vi "Progetto Sistemi Di Acquisizione Dati Urzino Davide.vi"() -> ()   [LabVIEW 2015]
uses:
  <vilib>/Instr/_visa.llb/VISA Configure Serial Port (Instr).vi
  <vilib>/smtpClient/Set Message Text.vi
  <vilib>/smtpClient/LabVIEWSMTPClient.lvlib
panel:
  in  "Invia Mail":bool
  in  "Percorso File":path
  out "ora corrente":string
  out "data corrente":string
  out "ora accensione":string
  out "data accensione":string
  out "Pulsante premuto":bool
  out "Contatore Pulsante":i32
  out "Grafico lettura fotodiodo":cluster{"Value":dbl, "Value":dbl}(graph)
  in  "stop":bool
  in  "Impostazione \nSoglia":dbl
  out "Soglia superata":bool
  out "Contatore Pezzi":i32
  out "Lettura bottone da seriale":string
  out "Lettura fotodiodo da seriale":dbl
  out "Minuto passato":bool
  # "Data e Ora di Start"
  # "Data e Ora Correnti"
  # "Imposta \nSoglia"
  # "Contatore Pezzi"
  # "Contatore Pulsante"
  # "Pulsante Premuto"
  # "Soglia Superata"
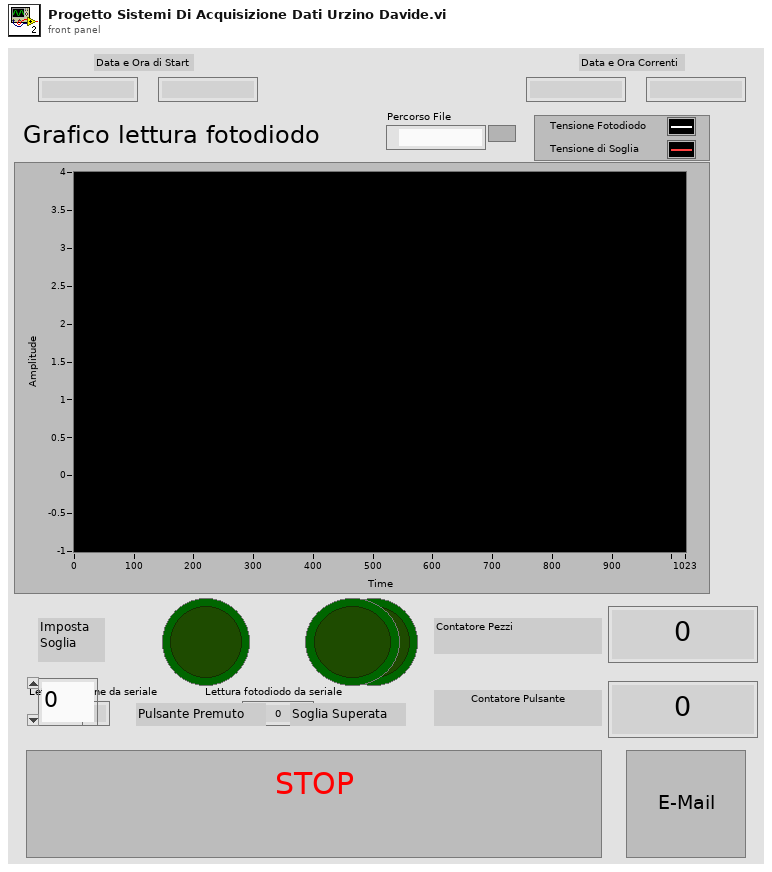
[diagram p1: front panel]
types:
  T1 = enum16{"open", "replace", "create", "open or create", "replace or create", "replace or create with confirmation"}
  T2 = typedef "LabVIEWSMTPClient.lvlib/SmtpClientHandle.ctl" = refnum<k1>
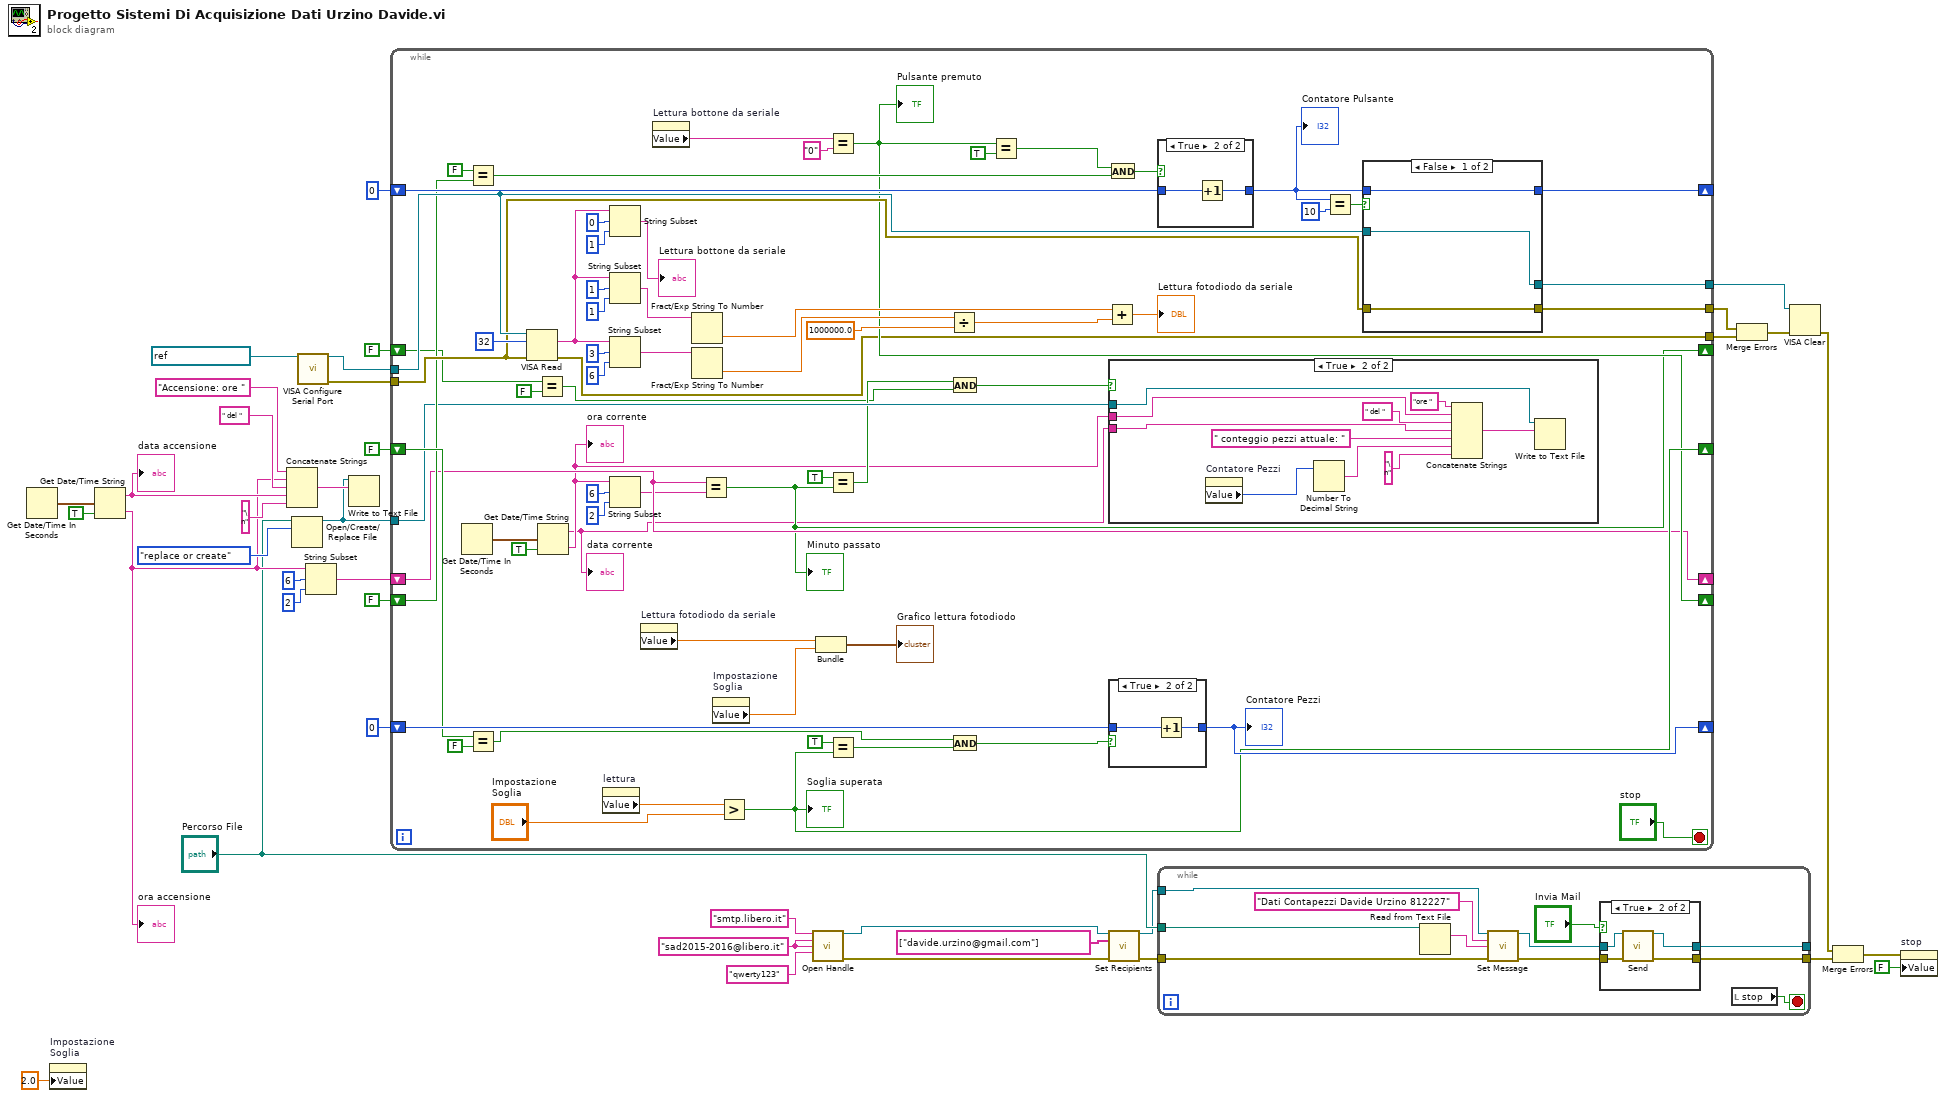
[diagram p0: block diagram]
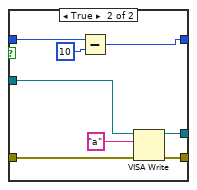
[diagram p4: hidden frame]
diagram:
  w7 = "sad2015-2016@libero.it" ("from")
  n1 = Get Date/Time In Seconds() -> (seconds since 1Jan1904=w31:timestamp)
  n2 = property on="Impostazione \nSoglia" class="DigNum (strict)"("Value"=2.0 ("Impostazione \nSoglia")) -> ()  [unwired: 2 in, 2 out]
  n3 = Get Date/Time String(seconds (now)=w31, want seconds? (F)=TRUE) -> (date string=w26:string, time string=w22:string)  [unwired: 1 in]
  "data accensione" <- w26
  "ora accensione" <- w22
  n4 = Concatenate Strings("Accensione: ore " ("string"), w22, " del " ("string"), w26, "\n" ("string")) -> (w29:string)
  n5 = Open/Create/Replace File(file path (use dialog)="Percorso File", operation (0:open)=T1."replace or create") -> (refnum out=w19:refnum<file>)  [unwired: 4 in, 2 out]
  n6 = call-poly "VISA Configure Serial Port"("VISA resource name"=refnum<visa-resource-name> "ASRL5::INSTR") -> ("VISA resource name out"=w39:refnum<visa-resource-name>, "error out"=w37:errorcluster)  [unwired: 13 in]
  n7 = String Subset(string=w22, offset (0)=6, length (rest)=2 ("length (rest)")) -> (substring=w21:string)
  n8 = Write to Text File(file (use dialog)=w19, text=w29) -> ()  [unwired: 2 in, 3 out]
  n9 = while {
    tunnel: w39 -> [w76]
    tunnel: w37 -> [w75]
    shift-right: [w73] -> _
    shift-left: 0 -> [w104]
    shift-right: [w70] -> _
    shift-left: FALSE -> [w72]
    shift-right: [w74] -> _
    shift-left: 0 -> [w79]
    shift-right: [w59] -> _
    shift-left: FALSE ("x") -> [w66]
    tunnel: w19 -> [w56]
    shift-right: [w53] -> _
    shift-left: w21 -> [w53]
    shift-right: [w45] -> _
    shift-left: FALSE ("want seconds? (F)") -> [w50]
    tunnel: [w42] -> w16
    tunnel: [w41] -> w15
    tunnel: [w40] -> w14
    stop <- "stop" stop-if-true
    n10 = Get Date/Time In Seconds() -> (seconds since 1Jan1904=w58:timestamp)
    n11 = Equal?(x=FALSE, y=w66) -> (x = y?=w62:bool)
    n12 = Equal?(x=w72, y=FALSE) -> (x = y?=w67:bool)
    n13 = VISA Read(VISA resource name=w76, byte count=u32 32, error in (no error)=w75) -> (read buffer=w83:string, error out=w41:errorcluster)  [unwired: 2 out]
    n14 = Equal?(x=w50, y=FALSE ("want seconds? (F)")) -> (x = y?=w47:bool)
    n15 = Get Date/Time String(seconds (now)=w58, want seconds? (F)=TRUE) -> (date string=w43:string, time string=w44:string)  [unwired: 1 in]
    "data corrente" <- w43
    "ora corrente" <- w44
    n16 = property on="lettura" class="DigNum (strict)"() -> ("Value"=w92:dbl)  [unwired: 2 in, 2 out]
    n17 = String Subset(string=w83, offset (0)=0, length (rest)=1 ("length (rest)")) -> (substring=→"Lettura bottone da seriale":string)
    n18 = String Subset(string=w83, offset (0)=1, length (rest)=1 ("length (rest)")) -> (substring=w102:string)
    n19 = String Subset(string=w83, offset (0)=3, length (rest)=6 ("length (rest)")) -> (substring=w100:string)
    n20 = String Subset(string=w44, offset (0)=6, length (rest)=2 ("length (rest)")) -> (substring=w52:string)
    n21 = property on="Lettura fotodiodo da seriale" class="DigNum (strict)"() -> ("Value"=w89:dbl)  [unwired: 2 in, 2 out]
    n22 = property on="Lettura bottone da seriale" class="Str"() -> ("Value"=w81:string)  [unwired: 2 in, 2 out]
    n23 = Fract/Exp String To Number(string=w102) -> (number=w97:dbl)  [unwired: 3 in, 1 out]
    n24 = Fract/Exp String To Number(string=w100) -> (number=w99:dbl)  [unwired: 3 in, 1 out]
    n25 = Equal?(x=w53, y=w52) -> (x = y?=w45:bool)
    "Minuto passato" <- w45
    n26 = property on="Impostazione \nSoglia" class="DigNum (strict)"() -> ("Value"=w88:dbl)  [unwired: 2 in, 2 out]
    n27 = Greater?(x=w92, y="Impostazione \nSoglia") -> (0:w70:bool)
    "Soglia superata" <- w70
    n28 = Bundle("Value"=w89, "Value"=w88) -> (→"Grafico lettura fotodiodo":cluster{"Value":dbl, "Value":dbl})  [unwired: 1 in]
    n29 = Equal?(x=w81, y="0") -> (x = y?=w59:bool)
    "Pulsante premuto" <- w59
    n30 = Equal?(x=TRUE, y=w45) -> (x = y?=w48:bool)
    n31 = Equal?(x=TRUE, y=w70) -> (x = y?=w68:bool)
    n32 = Divide(x=w99, y=1000000.0) -> (x/y=w96:dbl)
    n33 = And(x=w48, y=w47) -> (x .and. y?=w46:bool)
    n34 = And(x=w67, y=w68) -> (x .and. y?=w86:bool)
    n35 = Equal?(x=w59, y=TRUE) -> (x = y?=w63:bool)
    n36 = Add(x=w97, y=w96) -> (x+y=→"Lettura fotodiodo da seriale":dbl)
    n37 = And(x=w63, y=w62) -> (x .and. y?=w61:bool)
    n38 = case shown="True" w46 {
      tunnel: w56 -> [_ w115]
      tunnel: w44 -> [_ w112]
      tunnel: w43 -> [_ w110]
      frame False {
      }
      frame True {
        n39 = property on="Contatore Pezzi" class="DigNum (strict)"() -> ("Value"=w107:i32)  [unwired: 2 in, 2 out]
        n40 = Number To Decimal String(number=w107) -> (decimal integer string=w106:string)  [unwired: 1 in]
        n41 = Concatenate Strings("ore " ("string"), w112, " del " ("string"), w110, " conteggio pezzi attuale: " ("string"), w106, "\n" ("string")) -> (w114:string)
        n42 = Write to Text File(file (use dialog)=w115, text=w114) -> ()  [unwired: 2 in, 3 out]
      }
    }
    n43 = case shown="True" w86 {
      tunnel: w104 -> [w130 w132]
      tunnel: [w130 w131] -> w73
      frame False {
      }
      frame True {
        n44 = Increment(x=w132) -> (x+1=w131:i32)
      }
    }
    "Contatore Pezzi" <- w73
    n45 = case shown="True" w61 {
      tunnel: w79 -> [w127 w128]
      tunnel: [w127 w129] -> w60
      frame False {
      }
      frame True {
        n46 = Increment(x=w128) -> (x+1=w129:i32)
      }
    }
    "Contatore Pulsante" <- w60
    n47 = Equal?(x=w60, y=10) -> (x = y?=w78:bool)
    n48 = case shown="False" w78 {
      tunnel: w76 -> [w117 w123]
      tunnel: w75 -> [w116 w122]
      tunnel: w60 -> [w118 w126]
      tunnel: [w118 w125] -> w74
      tunnel: [w116 w120] -> w42
      tunnel: [w117 w119] -> w40
      frame False {
      }
      frame True {
        n49 = Subtract(x=w126, y=10) -> (x-y=w125:i32)
        n50 = VISA Write(VISA resource name=w123, write buffer="a", error in (no error)=w122) -> (VISA resource name out=w119:refnum<visa-resource-name>, error out=w120:errorcluster)  [unwired: 1 out]
      }
    }
  }
  n51 = call <vilib>:"Open Handle.vi"("server address"="smtp.libero.it", "from"=w7, "username"=w7, "password"="qwerty123") -> ("handle out"=w12:T2, "error out"=w11:errorcluster)  [unwired: 10 in]
  n52 = call <vilib>:"Set Recipients.vi"("handle in"=w12, "to"=string[] ["davide.urzino@gmail.com"], "error in (no error)"=w11) -> ("handle out"=w10:T2, "error out"=w9:errorcluster)  [unwired: 11 in]
  n53 = while {
    tunnel: [w137] -> w2
    tunnel: [w136] -> _
    tunnel: "Percorso File" -> [w135]
    tunnel: w10 -> [w134]
    tunnel: w9 -> [w133]
    stop <- w142 stop-if-true
    n54 = Read from Text File(file (use dialog)=w135) -> (text=w138:string)  [unwired: 3 in, 3 out]
    n55 = call-poly <vilib>:"Set Message.vi"("handle in"=w134, "subject"="Dati Contapezzi Davide Urzino 812227", "plain text message"=w138, "error in (no error)"=w133) -> ("handle out"=w140:T2, "error out"=w139:errorcluster)  [unwired: 10 in]
    n56 = case shown="True" "Invia Mail" {
      tunnel: w140 -> [w144 w149]
      tunnel: w139 -> [w145 w148]
      tunnel: [w145 w147] -> w137
      tunnel: [w144 w146] -> w136
      frame False {
      }
      frame True {
        n57 = call <vilib>:"Send.vi"("handle in"=w149, "error in (no error)"=w148) -> ("handle out"=w146:T2, "error out"=w147:errorcluster)  [unwired: 11 in, 1 out]
      }
    }
    n58 = local read "stop"() -> (w142:bool)
  }
  n59 = Merge Errors(w16, w15) -> (w17:errorcluster)
  n60 = VISA Clear(VISA resource name=w14, error in (no error)=w17) -> (error out=w3:errorcluster)  [unwired: 1 out]
  n61 = Merge Errors(w3, w2) -> (w1:errorcluster)
  n62 = property on="stop" class="Bool (strict)"(error in=w1, "Value"=FALSE ("stop")) -> ()  [unwired: 1 in, 2 out]
